vi "Broadcast.vi"(8 "error in (no error)":errorcluster, 10 "Data":string, 11 "WebSocket Service Actor in":refnum<class "WebSocket Service.lvclass">) -> (0 "error out":errorcluster, 3 "WebSocket Service Actor out":refnum<class "WebSocket Service.lvclass">)   [LabVIEW 2016, in "WebSocket Actors.lvlib" / "WebSocket Service.lvclass"]
doc: "Broadcasts data to all the connected clients"
uses:
  WebSocket Service.lvclass
  WebSocket Service.lvclass/WebSocket Service.ctl
  <vilib>/ActorFramework/Message Enqueuer/Message Enqueuer.lvclass
  WebSocket Connection Messages/Send to Peer Msg/Send to Peer Msg.lvclass
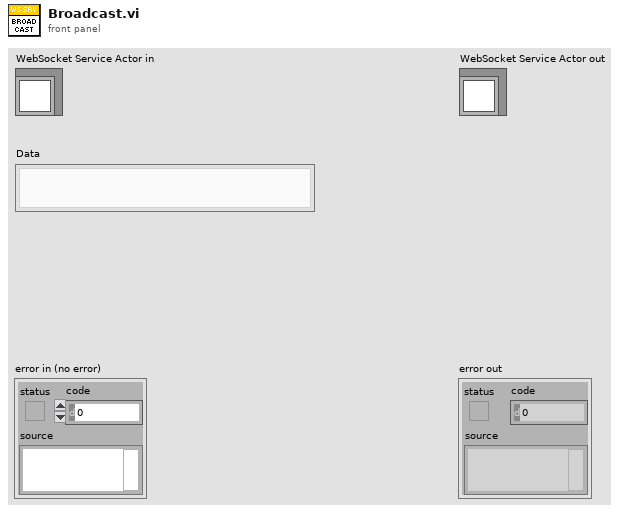
[diagram p1: front panel]
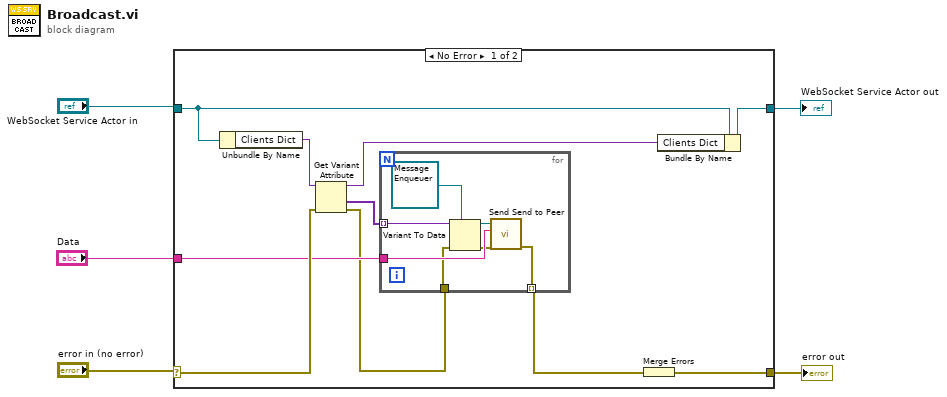
[diagram p0: block diagram]
diagram:
  n1 = case shown="No Error" "error in (no error)" {
    selector: "error in (no error)" -> [w12 w24]
    tunnel: [w6 w24] -> w1
    tunnel: [w14 w23] -> w3
    tunnel: "WebSocket Service Actor in" -> [w15 w23]
    tunnel: "Data" -> [w9 _]
    frame No Error {
      n2 = Unbundle By Name(w15) -> ("Clients Dict"=w13:variant)
      n3 = Get Variant Attribute(Variant=w13, error in=w12) -> (duplicate Variant=w11:variant, values=w10:variant[], error out=w8:errorcluster)  [unwired: 2 in, 1 out]
      n4 = for {
        tunnel: w10 -> [w22] mode=indexing
        tunnel: w9 -> [w21]
        tunnel: w8 -> [w20]
        tunnel: [w19] -> w7 mode=indexing
        n5 = Variant To Data(error in=w20, type=refnum<class "Message Enqueuer.lvclass"> refnum ("Message Enqueuer in"), Variant=w22) -> (data=w16:refnum<class "Message Enqueuer.lvclass">, error out=w18:errorcluster)
        n6 = call "Send Send to Peer.vi"("error in (no error)"=w18, "Data"=w21, "Message Enqueuer in"=w16) -> ("error out"=w19:errorcluster)  [unwired: 7 in, 1 out]
      }
      n7 = Merge Errors(w7) -> (w6:errorcluster)
      n8 = Bundle By Name(cluster=w15, "Clients Dict"=w11) -> (w14:refnum<class "WebSocket Service.lvclass">)
    }
    frame Error {
    }
  }
  "error out" <- w1
  "WebSocket Service Actor out" <- w3
